vi "Untitled 2.vi"() -> ()   [LabVIEW 2016]
panel:
  out "standard error":string
  out "standard output":string
  in  "command line":string
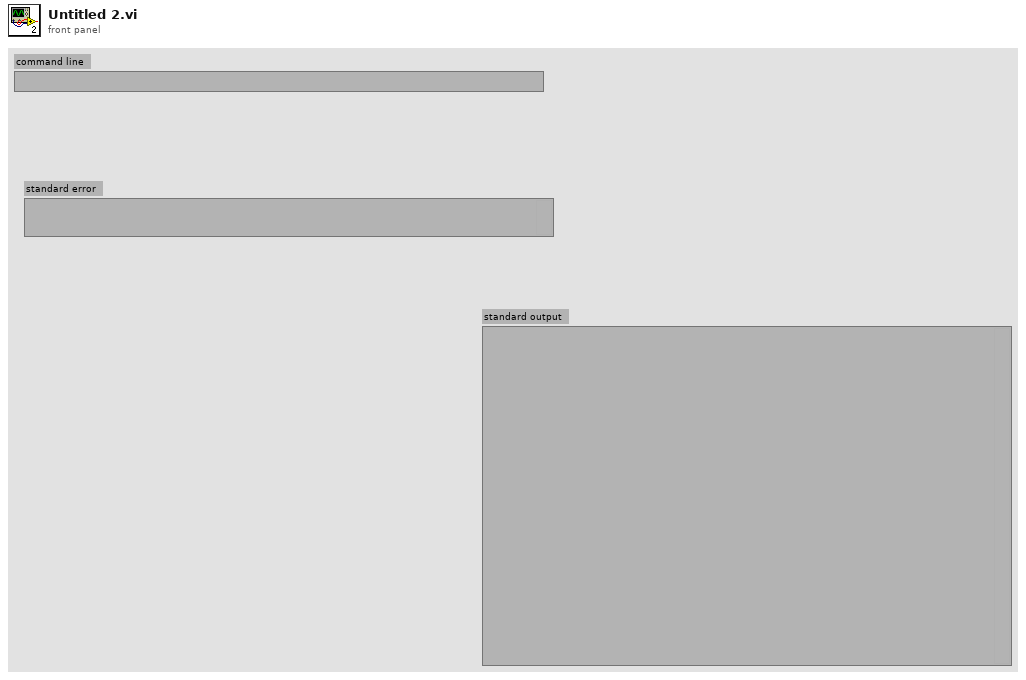
[diagram p1: front panel]
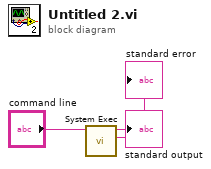
[diagram p0: block diagram]
diagram:
  n1 = call <vilib>:"System Exec.vi"("command line"="command line") -> ("standard error"=→"standard error":string, "standard output"=→"standard output":string)  [unwired: 7 in, 2 out]
